vi "Entity IDs.vi"(6 "Entity Manager in":refnum<class "Entity Manager.lvclass">, 11 "Entity Collection in":refnum<class "Entity Collection.lvclass">) -> (0 "error out":errorcluster, 2 "Entitiy IDs":T1[](array[typedef]), 3 "Entity Collection out":refnum<class "Entity Collection.lvclass">, 4 "Entity Manager":refnum<class "Entity Manager.lvclass">)   [LabVIEW 2020, in "Conditu2.lvlib" / "Columns.lvlib" / "Entity Collection.lvclass"]
uses:
  Entity Collection.lvclass
  Entity ID.ctl
  Entity Manager/Entity Manager.lvclass
  Entity Collection.lvclass/Entity Collection.ctl
  Entity/Entity.lvclass/Entity.ctl
  ID/ID.lvclass/ID.ctl
  ID/Get.vi
  Entity/Entity.lvclass
  Conditu2.lvlib
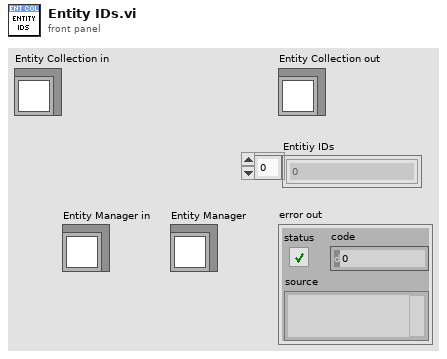
[diagram p1: front panel]
types:
  T1 = typedef "Conditu2.lvlib/Entity ID.ctl" = i64
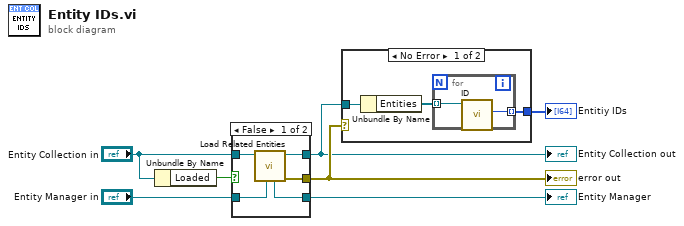
[diagram p0: block diagram]
diagram:
  n1 = Unbundle By Name("Entity Collection in") -> ("Loaded"=w7:bool)
  n2 = case shown="False" w7 {
    tunnel: "Entity Collection in" -> [w12 w13]
    tunnel: [w11 w13] -> w1
    tunnel: "Entity Manager in" -> [w10 w14]
    tunnel: [w9 w14] -> w4
    tunnel: [w8 _] -> w3
    frame False {
      n3 = call "Load Related Entities.vi"("Entity Manager in"=w10, "Entity Collection in"=w12) -> ("error out"=w8:errorcluster, "Entity Collection out"=w11:refnum<class "Entity Collection.lvclass">, "Entity Manager"=w9:refnum<class "Entity Manager.lvclass">)  [unwired: 7 in]
    }
    frame True {
    }
  }
  "Entity Manager" <- w4
  "Entity Collection out" <- w1
  "error out" <- w3
  n4 = case shown="No Error" w3 {
    tunnel: w1 -> [w17 _]
    tunnel: [w15 _] -> w2
    frame No Error {
      n5 = Unbundle By Name(w17) -> ("Entities"=w16:refnum<class "Entity.lvclass">[])
      n6 = for {
        tunnel: w16 -> [w19] mode=indexing
        tunnel: [w18] -> w15 mode=indexing
        n7 = call "ID.vi"("Entity in"=w19) -> ("ID"=w18:T1)  [unwired: 9 in, 1 out]
      }
    }
    frame Error {
    }
  }
  "Entitiy IDs" <- w2
